vi "HENES.vi"() -> ()   [LabVIEW 2024]
uses:
  <vilib>/Instr/_visa.llb/VISA Set IO Buffer Mask.ctl
  <vilib>/Instr/_visa.llb/VISA Flush IO Buffer Mask.ctl
  e33ea129-5426-40bd-9da2-e127971607b1.vi
  <vilib>/Instr/_visa.llb/VISA Configure Serial Port (Instr).vi
panel:
  out "GobackROI":cluster{i32[], i32[]}={[500, 500, -500, -500, 500], [100, 950, 950, 100, 100]}
  in  "Stop":bool
  in  "탭 컨트롤":enum32{"Main", "Debug"}(tab)
  in  "HLV_A/M":bool=TRUE
  out "Remote_M/A":bool
  out "E-STOP":bool=TRUE
  out "Alive_PCU":u8(slide)=1 scale=0.0..254.0
  out "Speed_Feed(RPM)":dbl format="%#_g rpm"
  in  "HLV_E-stop":bool
  out "Speed_Feed(m/s)":dbl
  in  "Input_Spd(kph)":dbl=7.0
  out "Input_Spd(cmd)":dbl=538.4742241275792
  in  "Lidar Tab":enum32{"Lidar", "Debug"}(tab)
  out "PointCloud":T1(graph)=[{"appended array"=[700.0, 700.0, 3500.0, 3500.0, -3500.0, -3500.0, -700.0, -700.0, 700.0], "appended array"=[800.0, -800.0, -800.0, 5200.0, 5200.0, -800.0, -800.0, 800.0, 800.0]}, {"appended array"=[-450.0], "appended array"=[-250.0]}, {"appended array"=[-450.0, -450.0, -800.0, -800.0, 0.0, 0.0, -450.0], "appended array"=[100.0, -800.0, -800.0, 1200.0, 1200.0, 100.0, 100.0]}, {"appended array"=[800.0, 750.0, 800.0, 800.0, 800.0, 800.0, 800.0], "appended array"=[400.0, 350.0, 350.0, 300.0, 250.0, 200.0, 150.0]}, {"appended array"=[450.0, 450.0, 800.0, 800.0, 0.0, 0.0, 450.0], "appended array"=[100.0, -800.0, -800.0, 1200.0, 1200.0, 100.0, 100.0]}, {"appended array"=array[442 elements], "appended array"=array[442 elements]}, {"appended array"=[4.2861222383783204e-13, 0.0], "appended array"=[7000.0, 0.0]}, {"appended array"=[500.0, 500.0, -500.0, -500.0, 500.0], "appended array"=[100.0, 950.0, 950.0, 100.0, 100.0]}]
  in  "격자크기":dbl=50.0
  out "LidarLoop":u32=101
  in  "Ratio_Threshold":i32=4
  in  "min_samples":i32=2
  in  "eps":i32=100
  in  "Spacing":i32=100
  in  "Threshold":i32=2100
  out "Too Close":bool=TRUE caption="lidar_state"
  in  "Looking Y":i32=5200
  in  "Looking X":i32=3500
  out "Anthena_Steer":i32
  out "NearSteer":dbl=28.559259641865033
  out "TooClose":bool=TRUE
  out "PythonLoop":u32=101
  in  "LiDAR":refnum<visa-resource-name>="COM5"
  in  "GoBack":bool
  out "VEstop":bool
  in  "length":dbl=1300.0
  out "read buffer":string
  out "Clustering Error":errorcluster
  in  "InputSteer(cmd)":dbl=28.559259641865033
  out "Steer_Feed":dbl=-0.28
  in  "HLV_Gear":u8
  out "Gear_Feed":u8=1
  out "HENES Loop Time":u32=48
  in  "HENES":refnum<visa-resource-name>="COM3"
  out "버퍼 읽기":string
  out "TargetDerection":cluster{dbl[], dbl[]}={[4.2861222383783204e-13, 0.0], [7000.0, 0.0]}
  out "NearLeft":dbl=77.70286898858113
  out "NearRight":dbl=-49.1436093467161
  out "Y_arraysREAL":i32[](array[numeric])=[1650, 1650, 1650, 1650, 1650, 1650, 1650, 1650, 1700, 1700, 1700, 1700, 1700, 1700, 1700, 1700, 1700, 1700, 1700, 1750, 1700]
  out "X_arraysREAL":i32[](array[numeric])=[1000, 1050, 1100, 1150, 1200, 1250, 1300, 1350, 1350, 1400, 1450, 1500, 1550, 1600, 1650, 1700, 1750, 1800, 1850, 1850, 1900]
  out "LookingAt":cluster{i32[], i32[]}={[700, 700, 3500, 3500, -3500, -3500, -700, -700, 700], [800, -800, -800, 5200, 5200, -800, -800, 800, 800]}
  out "Too Close":bool=TRUE caption="lidar_state"
  out "NearCarPointsRight":cluster{"ROI_IN_X":dbl[], "ROI_IN_Y":dbl[]}={"ROI_IN_X"=[750.0, 800.0, 800.0, 800.0, 800.0, 800.0], "ROI_IN_Y"=[350.0, 350.0, 300.0, 250.0, 200.0, 150.0]}
  out "NearCarROIRight":cluster{i32[], i32[]}={[450, 450, 800, 800, 0, 0, 450], [100, -800, -800, 1200, 1200, 100, 100]}
  out "Clustered":T2
  out "NearCarROILeft":cluster{i32[], i32[]}={[-450, -450, -800, -800, 0, 0, -450], [100, -800, -800, 1200, 1200, 100, 100]}
  out "NearCarPointsLeft":cluster{"ROI_IN_X":dbl[], "ROI_IN_Y":dbl[]}={"ROI_IN_X"=[-450.0, -550.0], "ROI_IN_Y"=[-250.0, -300.0]}
  out "Y_arrays":dbl[](array[numeric])=[1650.0, 1650.0, 1650.0, 1650.0, 1650.0, 1650.0, 1650.0, 1700.0, 1700.0, 1700.0, 1700.0, 1700.0, 1700.0, 1700.0, 1700.0, 1700.0, 1700.0, 1700.0, 1750.0, 1700.0, 1700.0, 1750.0, 1750.0, 1750.0, 1750.0, 1750.0, 1750.0, 1750.0, 1750.0, 1750.0, 1750.0, 1750.0, 1800.0, 1800.0, 1800.0, 1800.0, 1800.0, 1800.0, 1800.0, 1800.0, 1800.0, 1800.0, 1800.0, 1800.0, 1800.0, 1800.0, 1800.0, 1800.0, 1800.0, 1850.0, 1850.0, 1850.0, 350.0, 350.0, 350.0, 300.0, 250.0, 200.0, 200.0, 150.0, 150.0, 100.0, 50.0, 0.0, -50.0, -100.0, -150.0, -200.0, -250.0, -300.0, -300.0, -350.0, -400.0, -450.0, -500.0, -550.0, -600.0, -650.0, -700.0, -750.0, -800.0, -800.0, -750.0, -750.0, -700.0, -700.0, -650.0, -600.0, -550.0, -550.0, -500.0, -450.0, -400.0, -350.0, -300.0, -250.0, -200.0, -150.0, -100.0, -50.0, 0.0, 50.0, 100.0, 150.0, 200.0, 250.0, 300.0, 350.0, 400.0, 400.0, 450.0, 500.0, 550.0, 600.0, 600.0, 650.0, 650.0, 700.0, 700.0, 750.0, 750.0, 800.0, 800.0, 850.0, 850.0, 900.0, 900.0, 950.0, 950.0, 1000.0, 1000.0, 1050.0, 1050.0, 1100.0, 1100.0, 1150.0, 1150.0, 1200.0, 1200.0, 1250.0, 1250.0, 1300.0, 1300.0, 1350.0, 1400.0, 1450.0, 1500.0, 1550.0, 1600.0, 1650.0, 1700.0, 1750.0, 1800.0, 1850.0, 1900.0, 1950.0, 2000.0, 2050.0, 2100.0, 2150.0, 2200.0, 2250.0, 2300.0, 2350.0, 2400.0, 2450.0, 2500.0, 2550.0, 2600.0, 2600.0, 2650.0, 2700.0, 2750.0, 2800.0, 2850.0, 2900.0, 2950.0, 3000.0, 3050.0, 3100.0, 3150.0, 3200.0, 3250.0, 3300.0, 3350.0, 3400.0, 3450.0, 3450.0, 3500.0, 3550.0, 3600.0, 3650.0, 3700.0, 3750.0, 3800.0, 3850.0, 3900.0, 3950.0, 4000.0, 4000.0, 4100.0, 4150.0, 4200.0, 4250.0, 4300.0, 4350.0, 4400.0, 4450.0, 4500.0, 4550.0, 4600.0, 4650.0, 4700.0, 4750.0, 4800.0, 4900.0, 4950.0, 5000.0, 5050.0, 5100.0, 5150.0, 4500.0, 4500.0, 4600.0, 4550.0, 3800.0, 3700.0, 3650.0, 3600.0, 3550.0, 3500.0, 3500.0, 3450.0, 3400.0, 3350.0, 3300.0, 3250.0, 3250.0, 3200.0, 3150.0, 3200.0, 3200.0, 3200.0, 3400.0, 3450.0, 3200.0, 4700.0, 4700.0, 3700.0, 3450.0, 3400.0, 3450.0, 3500.0, 3500.0, 3450.0, 3400.0, 3400.0, 3350.0, 3300.0, 3300.0, 3250.0, 1600.0, 1600.0, 1650.0, 1600.0, 1650.0, 1735.0877192982457, -160.3448275862069, 1825.7462686567164, 5025.0, 4500.0, 4575.0, 3392.1052631578946, 3425.0, 4700.0, 3395.8333333333335, 1827.3513645224173, 1919.6150097465888, 2011.8786549707602, 2104.142300194932, 2196.4059454191033, 2288.669590643275, 2380.9332358674465, 2473.196881091618, 2565.4605263157896, 2657.7241715399614, 2749.9878167641327, 2842.251461988304, 2934.5151072124754, 3026.778752436647, 3119.042397660819, 3211.3060428849903, 3303.5696881091617, 1824.0304709141276, 1912.9732225300093, 2001.9159741458911, 2090.858725761773, 2179.801477377655, 2268.7442289935366, 2357.6869806094182, 2446.6297322253004, 2535.572483841182, 2624.5152354570637, 2713.457987072946, 2802.400738688827, 2891.343490304709, 2980.2862419205912, 3069.228993536473, 3158.1717451523546, 3247.114496768236, 3336.057248384118, 1817.938596491228, 1900.7894736842106, 1983.640350877193, 2066.4912280701756, 2149.342105263158, 2232.1929824561403, 2315.043859649123, 2397.8947368421054, 2480.745614035088, 2563.59649122807, 2646.4473684210525, 2729.2982456140353, 2812.149122807017, 2895.0, 2977.8508771929824, 3060.7017543859647, 3143.5526315789475, 3226.4035087719294, 3309.254385964912, 4515.0, 4530.0, 4545.0, 4560.0, 4407.675438596491, 4315.350877192983, 4223.026315789473, 4130.701754385965, 4038.377192982456, 3946.0526315789475, 3853.7280701754385, 3761.40350877193, 3669.078947368421, 3576.754385964912, 3484.4298245614036, 4417.307692307692, 4334.615384615385, 4251.923076923077, 4169.2307692307695, 4086.5384615384614, 4003.846153846154, 3921.153846153846, 3838.4615384615386, 3755.769230769231, 3673.076923076923, 3590.3846153846152, 3507.6923076923076, 4588.888888888889, 4602.777777777777, 4616.666666666667, 4630.555555555556, 4644.444444444444, 4658.333333333333, 4672.222222222223, 4686.111111111111, 4479.166666666667, 4383.333333333333, 4287.5, 4191.666666666667, 4095.8333333333335, 4000.0, 3904.166666666667, 3808.3333333333335, 3712.5, 3616.666666666667, 3520.8333333333335, 3403.0701754385964, 3414.035087719298, 3392.6378446115286, 3393.1704260651627, 3393.7030075187968, 3394.2355889724313, 3394.7681704260654, 3395.3007518796994, 3417.7083333333335, 3410.416666666667, 3403.125, 4684.615384615385, 4669.2307692307695, 4653.846153846154, 4638.461538461538, 4623.076923076923, 4607.692307692308, 4592.307692307692, 4576.923076923077, 4561.538461538462, 4546.153846153846, 4530.7692307692305, 4515.384615384615, 4606.8452380952385, 4513.690476190476, 4420.535714285715, 4327.380952380952, 4234.226190476191, 4141.071428571428, 4047.916666666667, 3954.761904761905, 3861.607142857143, 3768.452380952381, 3675.2976190476193, 3582.1428571428573, 3488.9880952380954, 3486.538461538462, 3577.24358974359, 3667.9487179487182, 3758.653846153846, 3849.3589743589746, 3940.0641025641025, 4030.769230769231, 4121.474358974359, 4212.179487179487, 4302.884615384615, 4393.589743589744, 4484.294871794872]
  out "X_arrays":dbl[](array[numeric])=[1050.0, 1100.0, 1150.0, 1200.0, 1250.0, 1300.0, 1350.0, 1350.0, 1400.0, 1450.0, 1500.0, 1550.0, 1600.0, 1650.0, 1700.0, 1750.0, 1800.0, 1850.0, 1850.0, 1900.0, 1950.0, 2000.0, 2050.0, 2100.0, 2150.0, 2200.0, 2250.0, 2300.0, 2350.0, 2400.0, 2450.0, 2500.0, 2500.0, 2550.0, 2600.0, 2650.0, 2700.0, 2750.0, 2800.0, 2850.0, 2900.0, 2950.0, 3000.0, 3050.0, 3100.0, 3150.0, 3200.0, 3250.0, 3300.0, 3350.0, 3400.0, 3450.0, 750.0, 800.0, 850.0, 800.0, 800.0, 800.0, 850.0, 800.0, 850.0, 850.0, 850.0, 850.0, 850.0, 850.0, 850.0, 850.0, 850.0, 850.0, 900.0, 900.0, 900.0, 900.0, 900.0, 900.0, 900.0, 900.0, 900.0, 900.0, 900.0, -2250.0, -2250.0, -2300.0, -2300.0, -2250.0, -2300.0, -2300.0, -2300.0, -2350.0, -2300.0, -2300.0, -2300.0, -2300.0, -2300.0, -2300.0, -2300.0, -2300.0, -2300.0, -2300.0, -2300.0, -2300.0, -2300.0, -2300.0, -2300.0, -2300.0, -2300.0, -2300.0, -2250.0, -2300.0, -2300.0, -2300.0, -2300.0, -2300.0, -2250.0, -2250.0, -2300.0, -2250.0, -2300.0, -2300.0, -2250.0, -2300.0, -2250.0, -2300.0, -2250.0, -2300.0, -2250.0, -2250.0, -2300.0, -2300.0, -2250.0, -2250.0, -2300.0, -2250.0, -2300.0, -2250.0, -2300.0, -2250.0, -2300.0, -2300.0, -2250.0, -2300.0, -2250.0, -2250.0, -2250.0, -2250.0, -2250.0, -2250.0, -2250.0, -2250.0, -2250.0, -2250.0, -2250.0, -2250.0, -2250.0, -2250.0, -2250.0, -2250.0, -2250.0, -2250.0, -2250.0, -2250.0, -2250.0, -2250.0, -2250.0, -2250.0, -2250.0, -2250.0, -2250.0, -2300.0, -2300.0, -2300.0, -2300.0, -2300.0, -2300.0, -2300.0, -2300.0, -2300.0, -2300.0, -2300.0, -2300.0, -2300.0, -2300.0, -2300.0, -2300.0, -2300.0, -2300.0, -2350.0, -2350.0, -2350.0, -2350.0, -2350.0, -2350.0, -2350.0, -2350.0, -2350.0, -2350.0, -2350.0, -2350.0, -2400.0, -2400.0, -2400.0, -2400.0, -2400.0, -2400.0, -2400.0, -2400.0, -2400.0, -2400.0, -2400.0, -2400.0, -2400.0, -2400.0, -2400.0, -2400.0, -2450.0, -2450.0, -2450.0, -2450.0, -2450.0, -2450.0, 650.0, 700.0, 1100.0, 1150.0, 950.0, 950.0, 950.0, 950.0, 950.0, 950.0, 1000.0, 1000.0, 1000.0, 1000.0, 1000.0, 1000.0, 1050.0, 1050.0, 1050.0, 1100.0, 1150.0, 1200.0, 1300.0, 1350.0, 1250.0, 1900.0, 1950.0, 1600.0, 1500.0, 1550.0, 1600.0, 1600.0, 1650.0, 1650.0, 1650.0, 1700.0, 1650.0, 1650.0, 1700.0, 1700.0, 900.0, 950.0, 950.0, 1000.0, 1000.0, 2118.4210526315787, 856.8965517241379, -2300.0, -2450.0, 675.0, 1125.0, 1028.9473684210527, 1325.0, 1925.0, 1633.3333333333333, 2091.4717348927875, 2064.522417153996, 2037.5730994152045, 2010.623781676413, 1983.6744639376216, 1956.7251461988303, 1929.7758284600388, 1902.8265107212474, 1875.877192982456, 1848.9278752436646, 1821.9785575048732, 1795.029239766082, 1768.0799220272904, 1741.130604288499, 1714.1812865497075, 1687.231968810916, 1660.2826510721247, 2076.6620498614957, 2034.9030470914126, 1993.1440443213294, 1951.3850415512463, 1909.6260387811633, 1867.8670360110802, 1826.108033240997, 1784.349030470914, 1742.590027700831, 1700.8310249307478, 1659.0720221606648, 1617.3130193905818, 1575.5540166204987, 1533.7950138504154, 1492.0360110803324, 1450.2770083102494, 1408.5180055401663, 1366.759002770083, 2063.9473684210525, 2009.4736842105262, 1954.9999999999998, 1900.5263157894735, 1846.0526315789473, 1791.5789473684208, 1737.1052631578946, 1682.6315789473683, 1628.157894736842, 1573.6842105263158, 1519.2105263157894, 1464.736842105263, 1410.2631578947367, 1355.7894736842104, 1301.3157894736842, 1246.842105263158, 1192.3684210526317, 1137.8947368421054, 1083.421052631579, 765.0, 855.0, 945.0, 1035.0, 704.4956140350878, 733.9912280701755, 763.4868421052631, 792.9824561403509, 822.4780701754387, 851.9736842105264, 881.469298245614, 910.9649122807018, 940.4605263157896, 969.9561403508773, 999.4517543859649, 725.0, 775.0, 825.0, 875.0, 925.0, 975.0, 1025.0, 1075.0, 1125.0, 1175.0, 1225.0, 1275.0, 1213.888888888889, 1302.7777777777778, 1391.6666666666665, 1480.5555555555557, 1569.4444444444443, 1658.3333333333333, 1747.2222222222222, 1836.111111111111, 1141.6666666666667, 1158.3333333333333, 1175.0, 1191.6666666666667, 1208.3333333333333, 1225.0, 1241.6666666666667, 1258.3333333333333, 1275.0, 1291.6666666666667, 1308.3333333333333, 1127.6315789473686, 1226.3157894736842, 1115.2882205513786, 1201.6290726817042, 1287.96992481203, 1374.310776942356, 1460.6516290726815, 1546.9924812030074, 1402.0833333333333, 1479.1666666666665, 1556.25, 1828.8461538461538, 1732.6923076923076, 1636.5384615384614, 1540.3846153846152, 1444.2307692307693, 1348.076923076923, 1251.9230769230767, 1155.7692307692307, 1059.6153846153848, 963.4615384615385, 867.3076923076922, 771.1538461538462, 1904.1666666666667, 1883.3333333333333, 1862.5, 1841.6666666666667, 1820.8333333333333, 1800.0, 1779.1666666666665, 1758.3333333333333, 1737.5, 1716.6666666666665, 1695.8333333333333, 1675.0, 1654.1666666666665, 1594.230769230769, 1555.128205128205, 1516.0256410256409, 1476.923076923077, 1437.8205128205127, 1398.7179487179487, 1359.6153846153845, 1320.5128205128203, 1281.4102564102564, 1242.3076923076924, 1203.2051282051282, 1164.102564102564]
  out "Y_arrays_input":i32[](array[numeric])=[1650, 1650, 1650, 1650, 1650, 1650, 1650, 1650, 1700, 1700, 1700, 1700, 1700, 1700, 1700, 1700, 1700, 1700, 1700, 1750, 1700]
  out "X_arrays_input":i32[](array[numeric])=[1000, 1050, 1100, 1150, 1200, 1250, 1300, 1350, 1350, 1400, 1450, 1500, 1550, 1600, 1650, 1700, 1750, 1800, 1850, 1850, 1900]
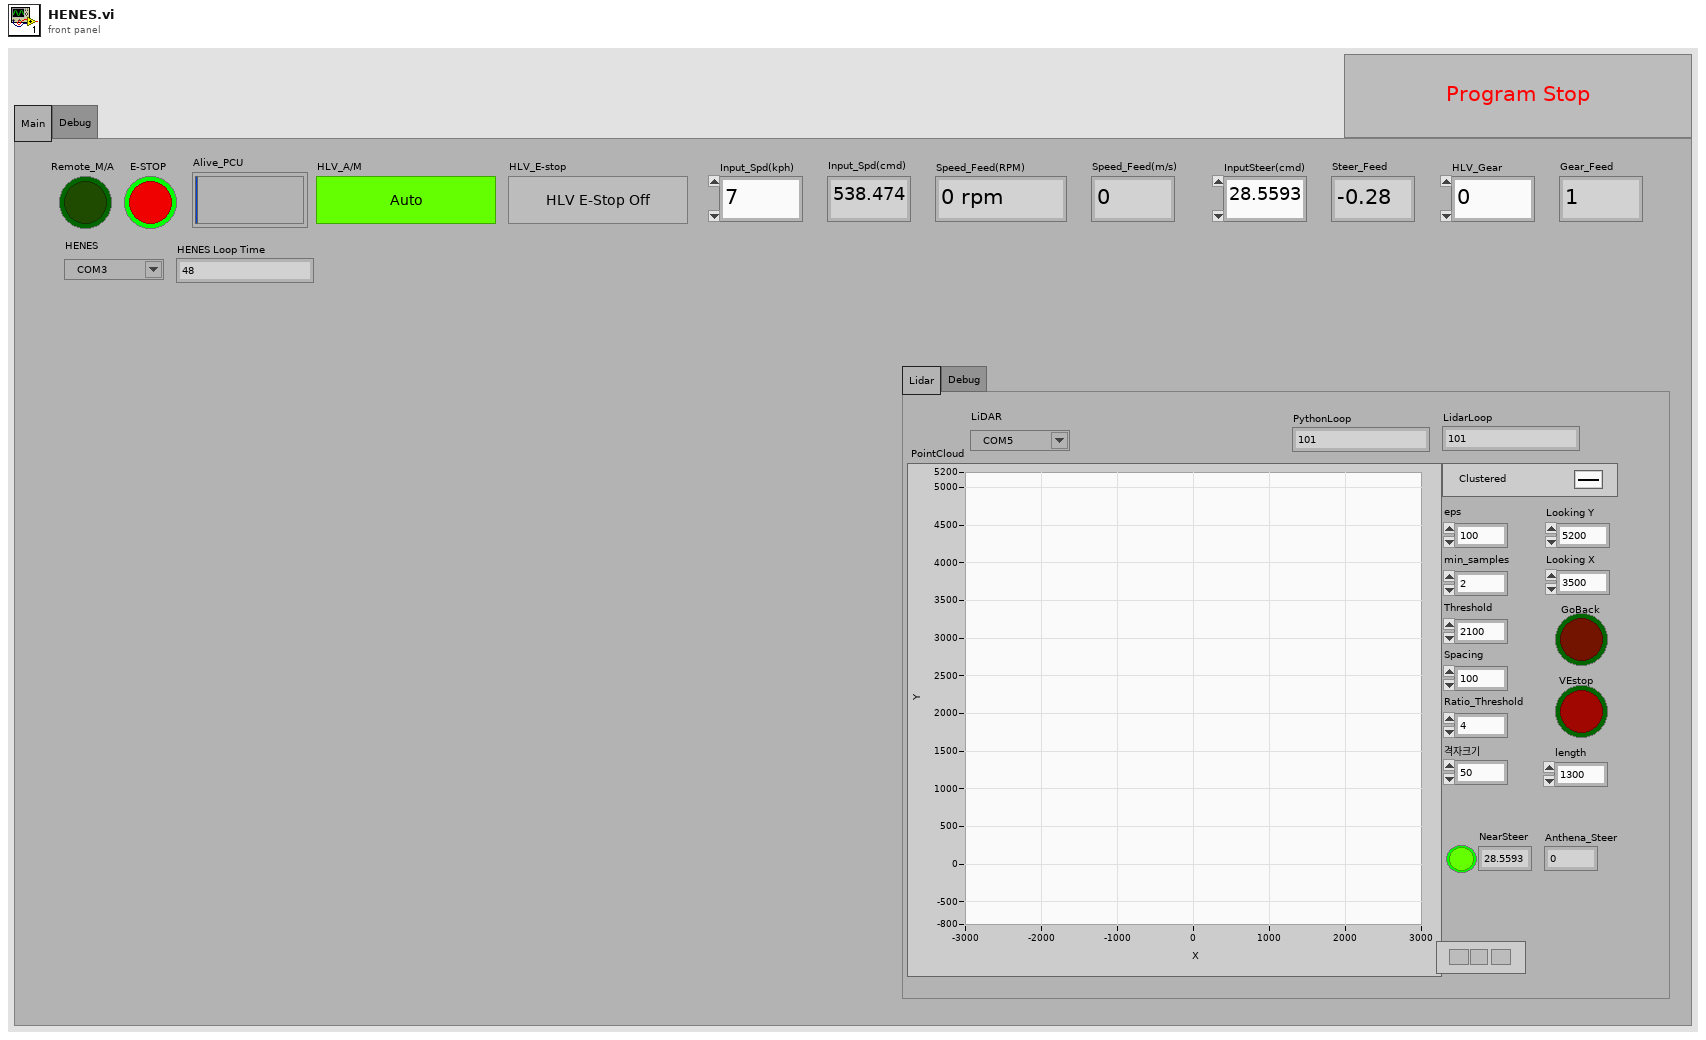
[diagram p1: front panel]
types:
  T1 = cluster{"appended array":dbl[], "appended array":dbl[]}[]
  T2 = cluster{"appended array":dbl[], "appended array":dbl[]}
  T3 = cluster{"HENES_M/A":u8, "HENES_E-Stop":u8, "HENES_Gear":u8, "HENES_Speed":i16, "HENES_Steer":i16, "HENES_Alive":u8}
  T4 = typedef "VISA Flush IO Buffer Mask.ctl" = u16
  T5 = typedef "VISA Set IO Buffer Mask.ctl" = u16
  T6 = cluster{"HLV_M/A_Status":u8, "HLV_E-Stop":u8, "HLV_Gear":u8, "HLV_Speed":i16, "HLV_Steer":i16, "HLV_Alive":u8}
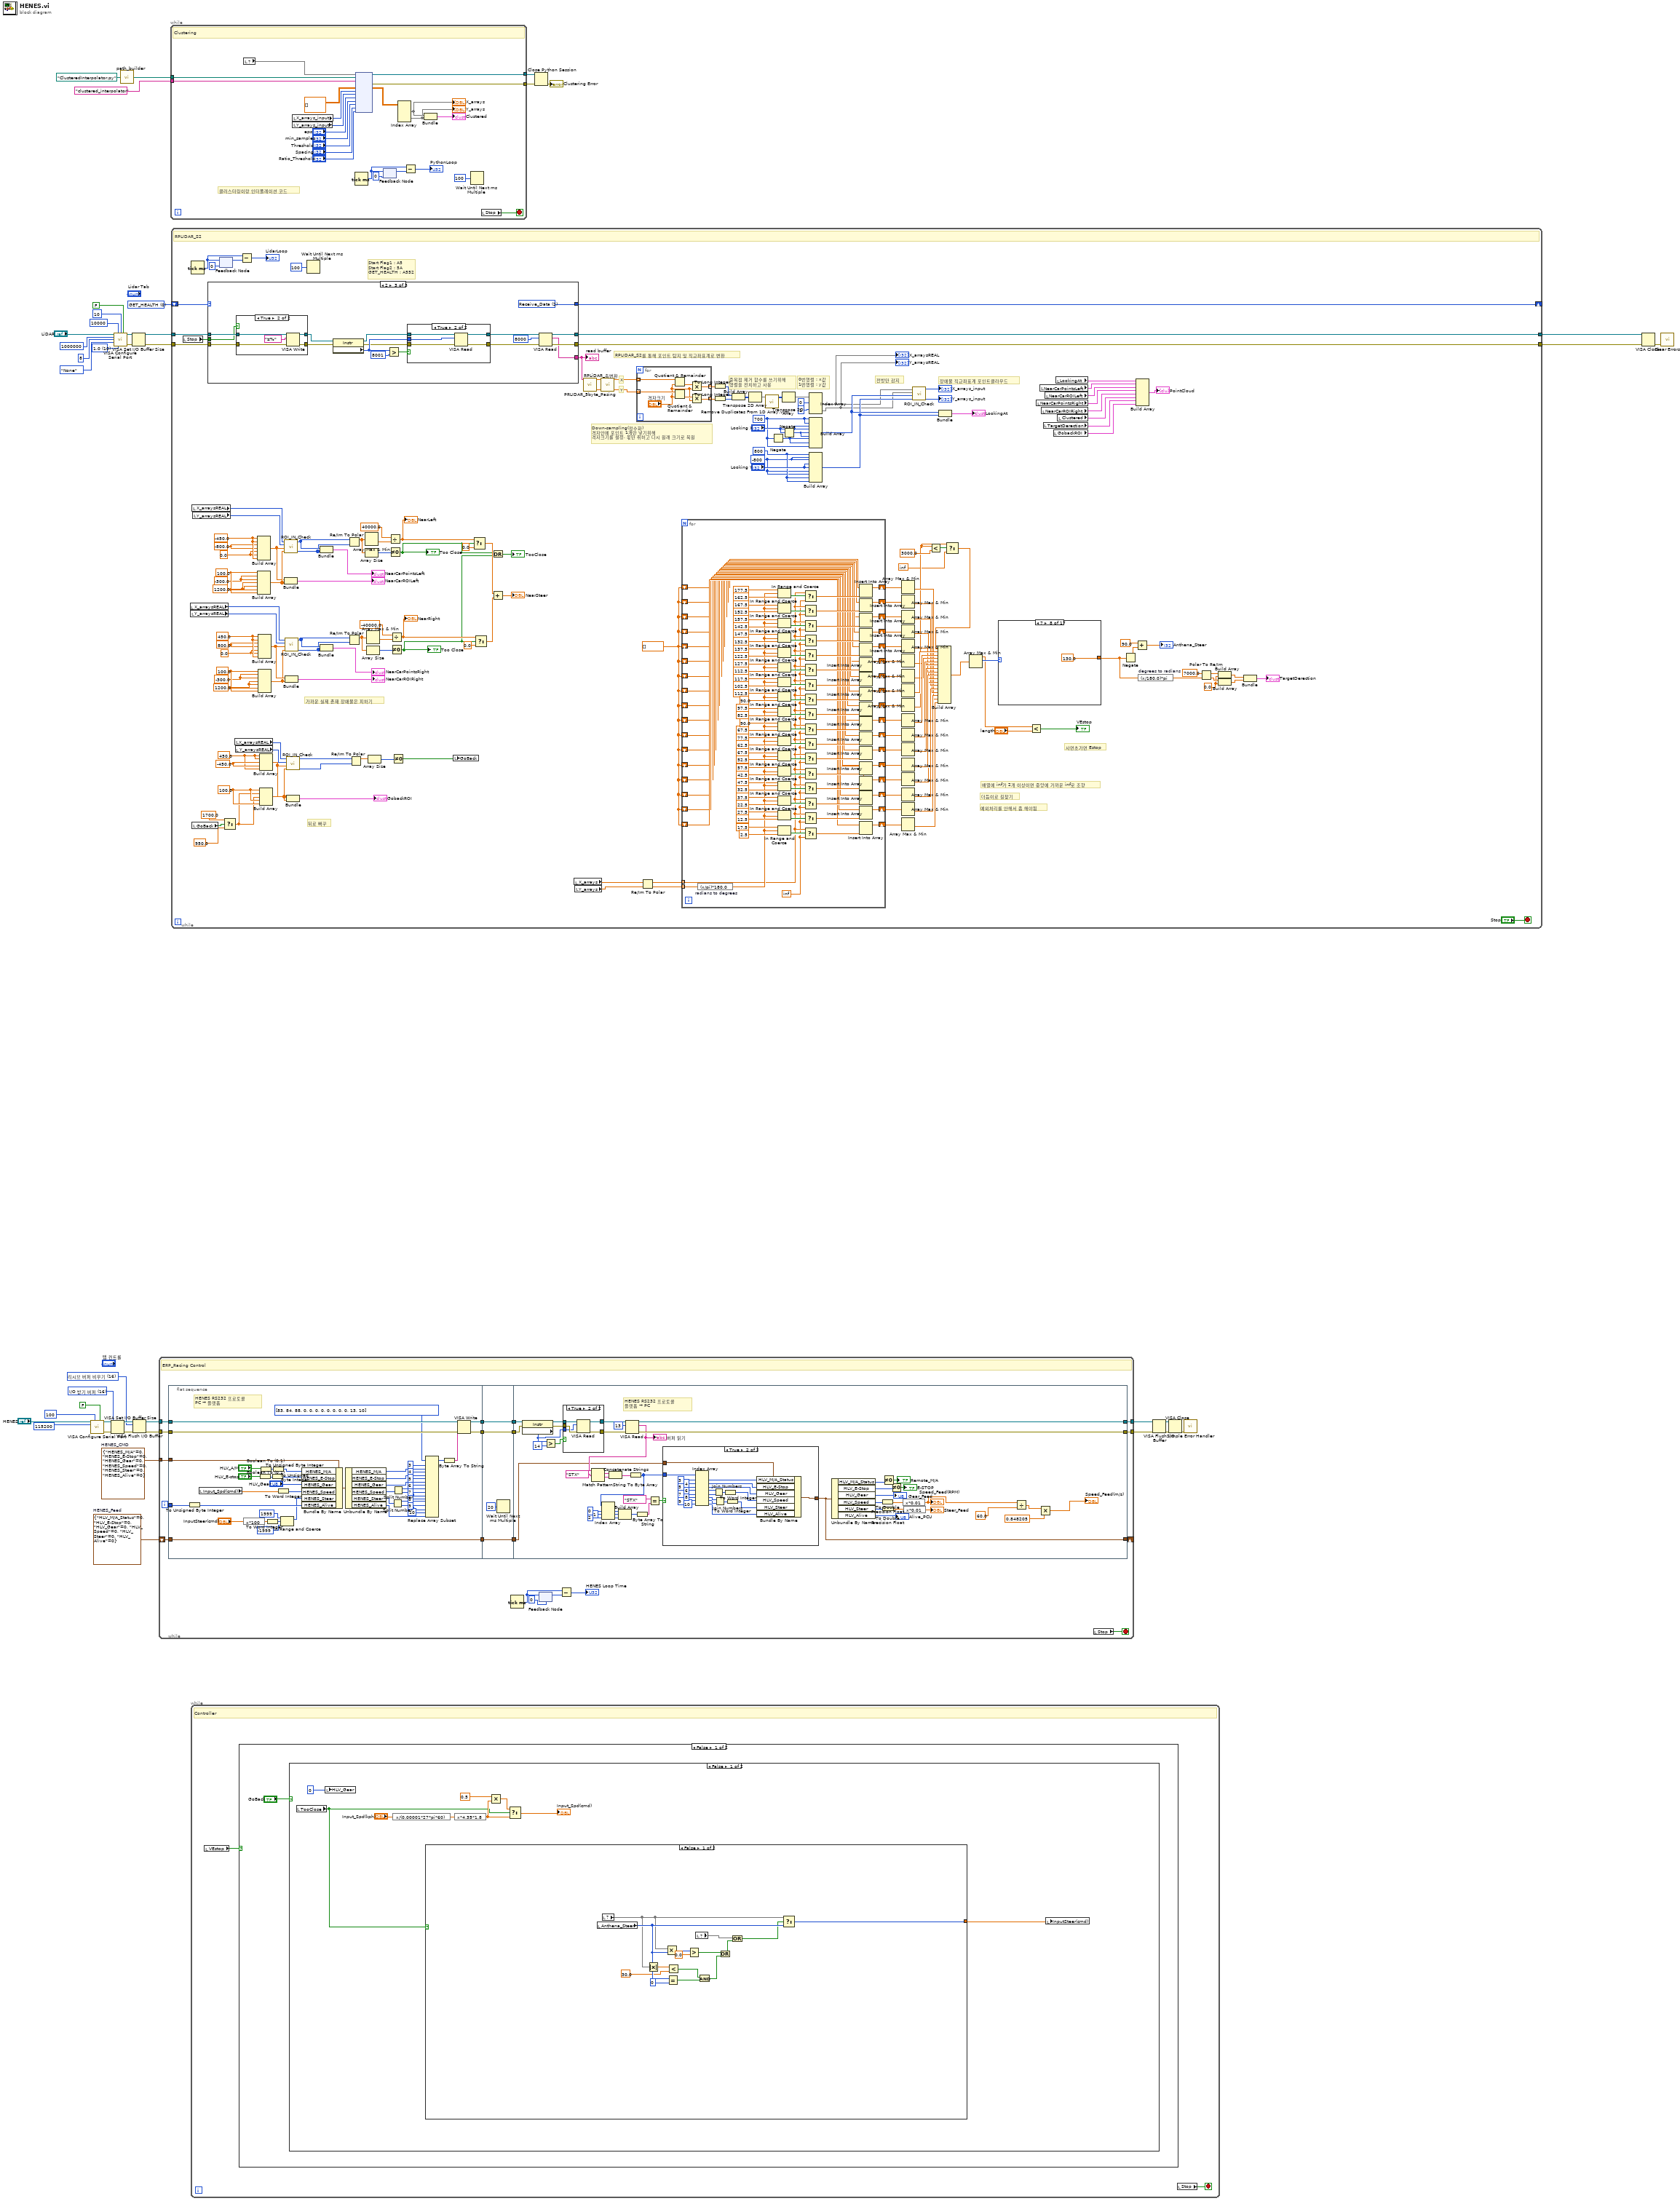
[diagram p0: block diagram]
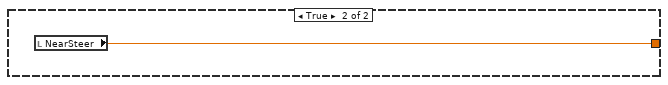
[diagram p2: hidden frame]
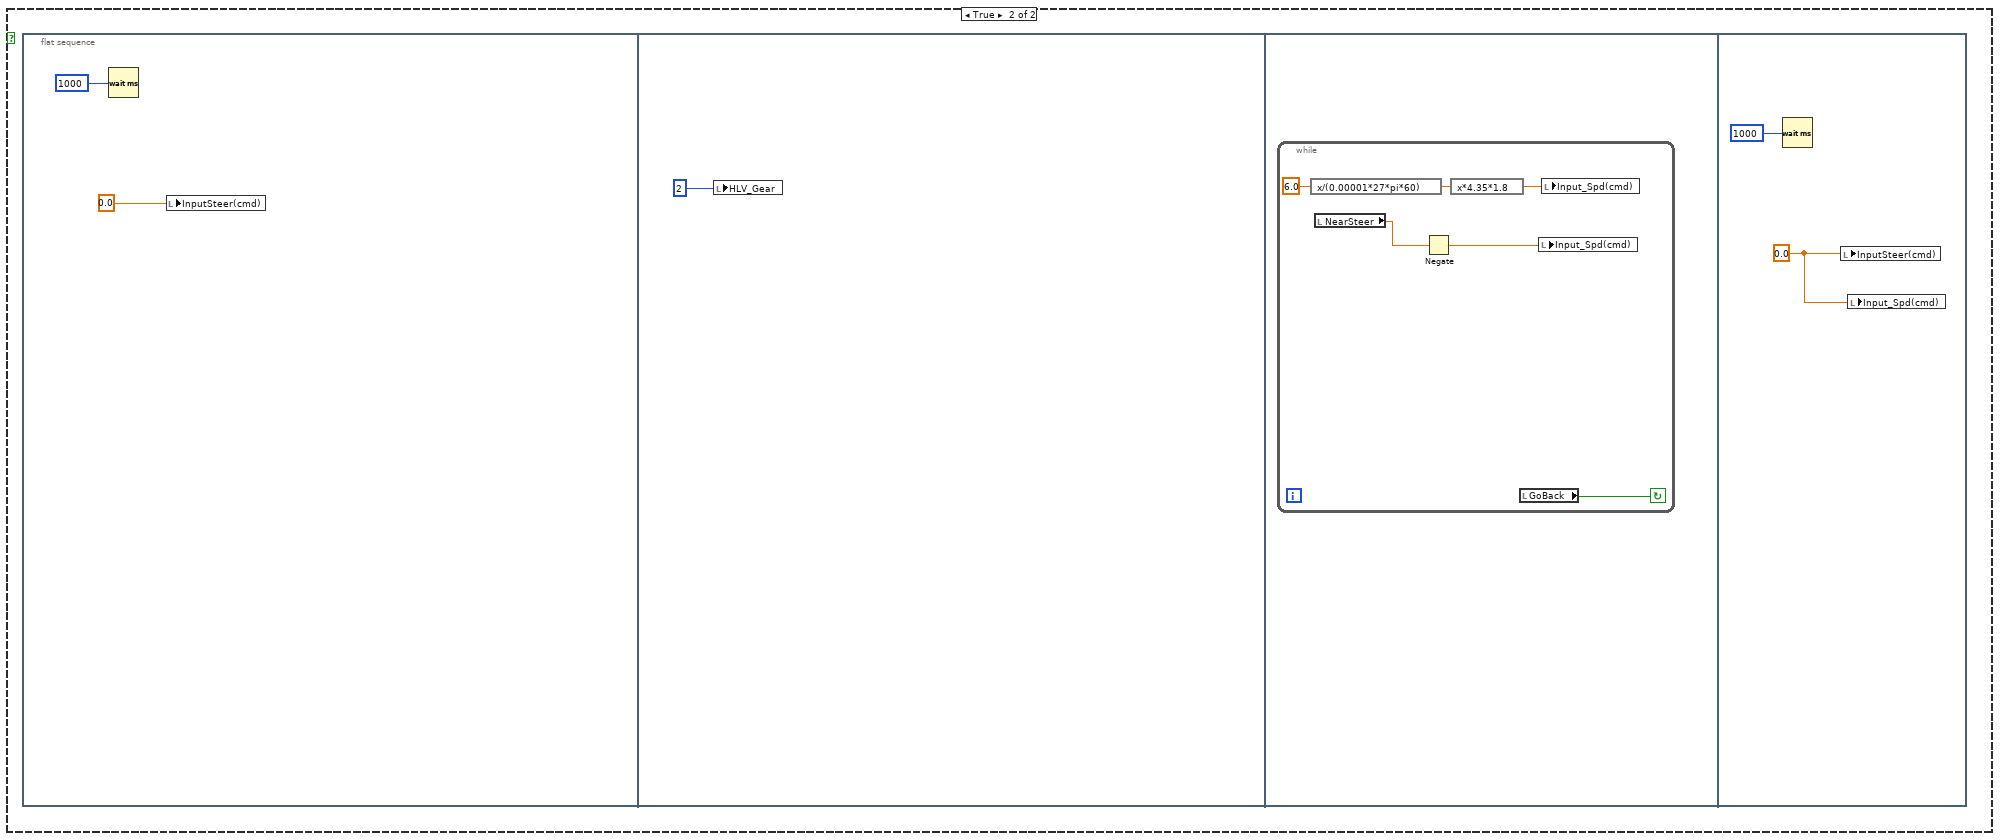
[diagram p3: hidden frame]
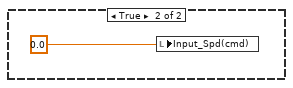
[diagram p4: hidden frame]
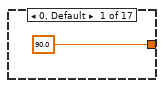
[diagram p7: hidden frame]
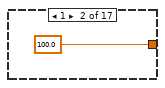
[diagram p8: hidden frame]
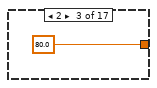
[diagram p9: hidden frame]
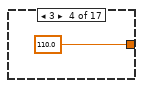
[diagram p10: hidden frame]
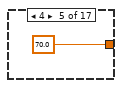
[diagram p11: hidden frame]
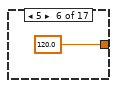
[diagram p12: hidden frame]
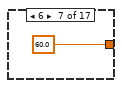
[diagram p13: hidden frame]
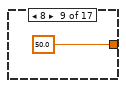
[diagram p14: hidden frame]
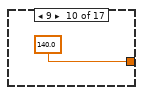
[diagram p15: hidden frame]
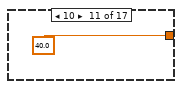
[diagram p16: hidden frame]
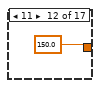
[diagram p17: hidden frame]
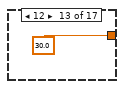
[diagram p18: hidden frame]
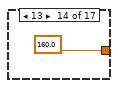
[diagram p19: hidden frame]
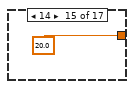
[diagram p20: hidden frame]
diagram:
  w3 = T3 {"HENES_M/A"=0, "HENES_E-Stop"=0, "HENES_Gear"=0, "HENES_Speed"=0, "HENES_Steer"=0, "HENES_Alive"=0}  # HENES_CMD
  w6 = T4 16 items=["리시브 버퍼 비우기"=16, "전달 버퍼 디바이스에 쓰기"=32, "리시브 버퍼 비우기(I/O 없음)"=64, "전달 버퍼 비우기"=128] ("Mask")
  w9 = T5 16 items=["I/O 받기 버퍼"=16, "I/O 전달 버퍼"=32, "I/O 받기와 전달 버퍼"=48] ("Mask")
  w13 = T6 {"HLV_M/A_Status"=0, "HLV_E-Stop"=0, "HLV_Gear"=0, "HLV_Speed"=0, "HLV_Steer"=0, "HLV_Alive"=0}  # HENES_Feed
  w27 = u16 10 items=["1.0"=10, "1.5"=15, "2.0"=20] ("stop bits (10: 1 bit)")
  w29 = u16 0 items=["GET_HEALTH", "SCAN_START", "Receive_Data"]
  n1 = call-poly "VISA Configure Serial Port"("VISA resource name"="HENES", "timeout (10sec)"=u32 100, "Enable Termination\nChar (T)"=FALSE ("Enable Termination\nChar (T)"), "baud rate (9600)"=u32 115200) -> ("VISA resource name out"=w5:refnum<visa-resource-name>, "error out"=w4:errorcluster)  [unwired: 10 in]
  n2 = VISA Set I/O Buffer Size(VISA resource name=w5, mask (16)=w9, error in (no error)=w4) -> (VISA resource name out=w8:refnum<visa-resource-name>, error out=w7:errorcluster)  [unwired: 1 in]
  n3 = call-poly "VISA Configure Serial Port"("VISA resource name"="LiDAR", "timeout (10sec)"=u32 10000, "termination char\n(0xA = '\\n' = LF)"=u8 10 ("termination char\n(0xA = '\\n' = LF)"), "Enable Termination\nChar (T)"=FALSE ("Enable Termination\nChar (T)"), "baud rate (9600)"=u32 1000000, "data bits (8)"=u16 8, "parity (0:none)"=enum16{"None", "Odd", "Even", "Mark", "Space"}."None", "stop bits (10: 1 bit)"=w27) -> ("VISA resource name out"=w36:refnum<visa-resource-name>, "error out"=w35:errorcluster)  [unwired: 6 in]
  n4 = call "path_builder.vi"("Name"=path "ClusteredInterpolator.py") -> ("appended path"=w22:path)
  n5 = VISA Set I/O Buffer Size(VISA resource name=w36, error in (no error)=w35) -> (VISA resource name out=w31:refnum<visa-resource-name>, error out=w30:errorcluster)  [unwired: 2 in]
  n6 = VISA Flush I/O Buffer(VISA resource name=w8, mask (16)=w6, error in (no error)=w7) -> (VISA resource name out=w18:refnum<visa-resource-name>, error out=w17:errorcluster)
  n7 = while {
    tunnel: w18 -> [w60]
    tunnel: w17 -> [w59]
    tunnel: [w53] -> w16
    tunnel: [w52] -> w15
    shift-right: [w47] -> _
    shift-left: w13 -> [w50]
    tunnel: w3 -> [w48]
    i -> [w54]
    stop <- w42 stop-if-true
    # "ERP_Racing Control"
    n8 = flat-sequence {
      tunnel: [w103] -> w57
      tunnel: [w102] -> w55
      tunnel: w60 -> [w105]
      tunnel: w59 -> [w104]
      tunnel: w54 -> [w101]
      tunnel: [w100] -> w51
      tunnel: w50 -> [w100]
      tunnel: w48 -> [w99]
      tunnel: [w109] -> w58
      tunnel: w57 -> [w109]
      tunnel: [w108] -> w56
      tunnel: w55 -> [w108]
      tunnel: w51 -> [w106]
      tunnel: [w106] -> w49
      tunnel: w58 -> [w137]
      tunnel: w56 -> [w136]
      tunnel: [w154] -> w53
      tunnel: [w153] -> w52
      tunnel: w49 -> [w128]
      tunnel: [w126] -> w47
      frame #0 {
        # "HENES RS232 프로토콜\nPC → 플랫폼"
        n9 = To Unsigned Byte Integer(number=w101) -> (unsigned 8bit integer=w88:u8)
        n10 = local read "Input_Spd(cmd)"() -> (w62:dbl)
        n11 = expression code="x*100"("InputSteer(cmd)") -> (w63:dbl)
        n12 = Boolean To (0,1)(Boolean="HLV_E-stop") -> (0, 1=w83:i16)
        n13 = Boolean To (0,1)(Boolean="HLV_A/M") -> (0, 1=w84:i16)
        n14 = To Word Integer(number=w63) -> (16bit integer=w66:i16)
        n15 = To Unsigned Byte Integer(number=w83) -> (unsigned 8bit integer=w81:u8)
        n16 = To Unsigned Byte Integer(number=w84) -> (unsigned 8bit integer=w82:u8)
        n17 = To Word Integer(number=w62) -> (16bit integer=w75:i16)
        n18 = In Range and Coerce(upper limit=i16 1999 ("상위 리미트"), x=w66, lower limit=i16 -1999 ("상위 리미트")) -> (coerced(x)=w74:i16)  [unwired: 1 out]
        n19 = Bundle By Name(cluster=w99, "HENES_M/A"=w82, "HENES_E-Stop"=w81, "HENES_Gear"="HLV_Gear", "HENES_Speed"=w75, "HENES_Steer"=w74, "HENES_Alive"=w88) -> (w92:T3)
        n20 = Unbundle By Name(w92) -> ("HENES_M/A"=w78:u8, "HENES_E-Stop"=w77:u8, "HENES_Gear"=w67:u8, "HENES_Speed"=w70:i16, "HENES_Steer"=w73:i16, "HENES_Alive"=w87:u8)
        n21 = Split Number(x=w73) -> (hi(x)=w72:u8, lo(x)=w71:u8)
        n22 = Split Number(x=w70) -> (hi(x)=w69:u8, lo(x)=w68:u8)
        n23 = Replace Array Subset(array=u8[] [83, 84, 88, 0, 0, 0, 0, 0, 0, 0, 0, 13, 10] ("unsigned byte array"), new element #1=w78, index #1=3, new element #2=w77, index #2=4, new element #3=w67, index #3=5, new element #4=w69, index #4=6, new element #5=w68, index #5=7, new element #6=w72, index #6=8, new element #7=w71, index #7=9, new element #8=w87, index #8=10) -> (w90:u8[])
        n24 = Byte Array To String(unsigned byte array=w90) -> (string=w89:string)
        n25 = VISA Write(VISA resource name=w105, write buffer=w89, error in (no error)=w104) -> (VISA resource name out=w103:refnum<visa-resource-name>, error out=w102:errorcluster)  [unwired: 1 out]
      }
      frame #1 {
        n26 = Wait Until Next ms Multiple(millisecond multiple=u32 20 ("대기 시간 (ms)")) -> ()  [unwired: 1 out]
      }
      frame #2 {
        # "HENES RS232 프로토콜\n플랫폼 → PC"
        n27 = property class="Instr"(reference=w137, error in=w136) -> (reference out=w117:refnum<visa-resource-name>, error out=w116:errorcluster, "Serial Settings:Number of Bytes at Serial Port"=w115:u32)
        n28 = Greater?(x=w115, y=u32 14) -> (0:w133:bool)
        n29 = case shown="True" w133 {
          tunnel: w117 -> [w181 w186]
          tunnel: w116 -> [w180 w185]
          tunnel: [w181 w184] -> w135
          tunnel: [w180 w183] -> w134
          tunnel: w115 -> [_ w182]
          frame False {
          }
          frame True {
            n30 = VISA Read(VISA resource name=w186, byte count=w182, error in (no error)=w185) -> (VISA resource name out=w184:refnum<visa-resource-name>, error out=w183:errorcluster)  [unwired: 2 out]
          }
        }
        n31 = VISA Read(VISA resource name=w135, byte count=u32 13, error in (no error)=w134) -> (VISA resource name out=w154:refnum<visa-resource-name>, read buffer=w152:string, error out=w153:errorcluster)  [unwired: 1 out]
        "버퍼 읽기" <- w152
        n32 = Match Pattern(string=w152, regular expression="STX") -> (match substring=w149:string, after substring=w150:string)  [unwired: 1 in, 2 out]
        n33 = Concatenate Strings(w149, w150) -> (w148:string)
        n34 = String To Byte Array(string=w148) -> (unsigned byte array=w130:u8[])
        n35 = Index Array(array=w130, index #1=0, index #2=1, index #3=2) -> (element #1=w143:u8, element #2=w142:u8, element #3=w141:u8)
        n36 = Build Array(w143, w142, w141) -> (w140:u8[])
        n37 = Byte Array To String(unsigned byte array=w140) -> (string=w138:string)
        n38 = Equal?(x="STX", y=w138) -> (x = y?=w129:bool)
        n39 = case shown="True" w129 {
          tunnel: w130 -> [_ w179]
          tunnel: [w156 w166] -> w126
          tunnel: w128 -> [w156 w168]
          frame False {
          }
          frame True {
            n40 = Index Array(array=w179, index #1=3, index #2=4, index #3=5, index #4=6, index #5=7, index #6=8, index #7=9, index #8=10) -> (element #1=w167:u8, element #2=w165:u8, element #3=w164:u8, element #4=w163:u8, element #5=w162:u8, element #6=w160:u8, element #7=w159:u8, element #8=w157:u8)
            n41 = Join Numbers(hi=w163, lo=w162) -> ((hi.lo)=w170:u16)
            n42 = Join Numbers(hi=w160, lo=w159) -> ((hi.lo)=w169:u16)
            n43 = To Word Integer(number=w170) -> (16bit integer=w161:i16)
            n44 = To Word Integer(number=w169) -> (16bit integer=w158:i16)
            n45 = Bundle By Name(cluster=w168, "HLV_M/A_Status"=w167, "HLV_E-Stop"=w165, "HLV_Gear"=w164, "HLV_Speed"=w161, "HLV_Steer"=w158, "HLV_Alive"=w157) -> (w166:T6)
          }
        }
        n46 = Unbundle By Name(w126) -> ("HLV_M/A_Status"=w127:u8, "HLV_E-Stop"=w121:u8, "HLV_Gear"=→"Gear_Feed":u8, "HLV_Speed"=w119:i16, "HLV_Steer"=w118:i16, "HLV_Alive"=→"Alive_PCU":u8)
        n47 = To Double Precision Float(number=w119) -> (double precision float=w131:dbl)
        n48 = To Double Precision Float(number=w118) -> (double precision float=w124:dbl)
        n49 = Not Equal To 0?(x=w127) -> (x != 0?=→"Remote_M/A":bool)
        n50 = Not Equal To 0?(x=w121) -> (x != 0?=→"E-STOP":bool)
        n51 = expression code="x*0.01"(w131) -> (w110:dbl)
        "Speed_Feed(RPM)" <- w110
        n52 = expression code="x*0.01"(w124) -> (→"Steer_Feed":dbl)
        n53 = Divide(x=w110, y=60.0) -> (x/y=w114:dbl)
        n54 = Multiply(x=w114, y=0.848205) -> (x*y=→"Speed_Feed(m/s)":dbl)
      }
    }
    n55 = Tick Count (ms)() -> (millisecond timer value=w44:u32)
    n56 = feedback #1(u32 0 ("millisecond timer value")) -> (w45:u32)
    n57 = feedback-in #1(w44) -> ()
    n58 = Subtract(x=w44, y=w45) -> (x-y=→"HENES Loop Time":u32)
    n59 = local read "Stop"() -> (w42:bool)
  }
  n60 = while {
    tunnel: w22 -> [w208]
    tunnel: "clustered_interpolator" ("function name") -> [w207]
    tunnel: [w206] -> w25
    tunnel: [w205] -> w26
    stop <- w209 stop-if-true
    # "클러스터링이랑 인터폴레이션 코드"
    # "Clustering"
    n61 = local read item#-1() -> (w187)
    n62 = local read "X_arrays_input"() -> (w204:i32[])
    n63 = local read "Y_arrays_input"() -> (w203:i32[])
    n64 = Tick Count (ms)() -> (millisecond timer value=w188:u32)
    n65 = node(w187, w208, w207, dbl[][] [] ("appended array"), w204, w203, "eps", "min_samples", "Threshold", "Spacing", "Ratio_Threshold") -> (w206:refnum<k35>, w205:errorcluster, w202:dbl[][])  [unwired: 8 in, 2 out]
    n66 = feedback #2(u32 0 ("millisecond timer value")) -> (w189:u32)
    n67 = feedback-in #2(w188) -> ()
    n68 = Index Array(array=w202) -> (element #1=w195:dbl[], element #2=w194:dbl[])  [unwired: 4 in]
    "X_arrays" <- w195
    "Y_arrays" <- w194
    n69 = Subtract(x=w188, y=w189) -> (x-y=→"PythonLoop":u32)
    n70 = Bundle("appended array"=w195, "appended array"=w194) -> (→"Clustered":T2)  [unwired: 1 in]
    n71 = Wait Until Next ms Multiple(millisecond multiple=u32 100) -> ()  [unwired: 1 out]
    n72 = local read "Stop"() -> (w209:bool)
  }
  n73 = while {
    tunnel: [w373] -> w40
    tunnel: [w374] -> w39
    tunnel: w31 -> [w382]
    tunnel: w30 -> [w381]
    shift-right: [w380] -> _
    shift-left: w29 -> [w383]
    stop <- "Stop" stop-if-true
    w238 = -450.0 ("element")
    w226 = 100.0 ("element")
    w228 = 450.0 ("element")
    w239 = 1200.0 ("f")
    w241 = 1200.0 ("element")
    w250 = dbl[] []
    w273 = 0.0 ("r")
    w309 = 0.0 ("element")
    w307 = -300.0 ("element")
    w310 = 800.0 ("element")
    w308 = 100.0 ("element")
    w311 = 450.0 ("element")
    w314 = 0.0 ("element")
    w312 = -300.0 ("element")
    w315 = -800.0 ("element")
    w313 = 100.0 ("element")
    w316 = -450.0 ("element")
    w349 = -800
    w350 = 800
    w351 = 700
    # "뒤로 빠꾸"
    # "사면초가면 Estop"
    # "배열에 inf가 2개 이상이면 중앙에 가까운 inf로 조향"
    # "예외처리를 안해서 좀 해야됨"
    # "더듬이로 길찾기"
    # "가까운 실제 존재 장애물은 피하기"
    # "전방만 감지"
    # "장애물 직교좌표계 포인트클라우드"
    # "RPLIDAR_S2를 통해 포인트 탐지 및 직교좌표계로 변환"
    # "Start Flag1 : A5\nStart Flag2 : 5A \nGET_HEALTH : A552"
    # "0번행렬 : x값\n1번행렬 : y값"
    # "중복점 제거 함수를 쓰기위해\n행렬을 전치하고 사용"
    # "Down-sampling(정수화)\n격자안에 포인트 1개만 넣기위해\n격자크기를 설정, 몫만 취하고 다시 원래 크기로 복원"
    # "Y"
    # "X"
    # "RPLIDAR_S2"
    n74 = local read "Stop"() -> (w379:bool)
    n75 = local read "X_arraysREAL"() -> (w216:i32[])
    n76 = local read "Y_arraysREAL"() -> (w215:i32[])
    n77 = Tick Count (ms)() -> (millisecond timer value=w378:u32)
    n78 = local read "X_arraysREAL"() -> (w217:i32[])
    n79 = local read "GoBack"() -> (w222:bool)
    n80 = local read "Y_arraysREAL"() -> (w218:i32[])
    n81 = case shown="2" w383 {
      tunnel: w382 -> [w531 w549 w572]
      tunnel: w381 -> [w530 w548 w571]
      tunnel: [w532 w545 w558] -> w380
      tunnel: [w521 w546 w574] -> w374
      tunnel: [w520 w547 w573] -> w373
      tunnel: w379 -> [_ _ w570]
      tunnel: ["" ("read buffer") w543 w569] -> w358
      frame 0, Default {
        w514 = u16 0 items=["GET_HEALTH", "SCAN_START", "Receive_Data"]
        w515 = u16 1 items=["GET_HEALTH", "SCAN_START", "Receive_Data"]
        n82 = VISA Write(VISA resource name=w531, write buffer="¥R", error in (no error)=w530) -> (VISA resource name out=w525:refnum<visa-resource-name>, error out=w524:errorcluster)  [unwired: 1 out]
        n83 = flat-sequence {
          tunnel: w525 -> [w534]
          tunnel: w524 -> [w533]
          tunnel: [w534] -> w523
          tunnel: [w533] -> w522
          frame #0 {
            n84 = Wait (ms)(milliseconds to wait=u32 5 ("대기 시간 (ms)")) -> ()  [unwired: 1 out]
          }
        }
        n85 = property class="Instr"(reference=w523, error in=w522) -> (reference out=w528:refnum<visa-resource-name>, error out=w527:errorcluster, "Serial Settings:Number of Bytes at Serial Port"=w526:u32)
        n86 = VISA Read(VISA resource name=w528, byte count=w526, error in (no error)=w527) -> (VISA resource name out=w520:refnum<visa-resource-name>, read buffer=w517:string, error out=w521:errorcluster)  [unwired: 1 out]
        n87 = Equal?(x=w517, y="¥Z\u0003\u0000\u0000\u0000\u0006\u0000\u0000\u0000") -> (x = y?=w518:bool)
        n88 = Select(t=w515, s=w518, f=w514) -> (s? t:f=w532:u16)
      }
      frame 1 {
        w536 = u16 2 items=["GET_HEALTH", "SCAN_START", "Receive_Data"]
        w537 = u16 1 items=["GET_HEALTH", "SCAN_START", "Receive_Data"]
        w550 = "¥Z\u0005\u0000\u0000@"
        n89 = VISA Write(VISA resource name=w549, write buffer="¥ \u0000", error in (no error)=w548) -> (VISA resource name out=w552:refnum<visa-resource-name>, error out=w553:errorcluster)  [unwired: 1 out]
        n90 = flat-sequence {
          tunnel: w552 -> [w556]
          tunnel: w553 -> [w555]
          tunnel: [w556] -> w539
          tunnel: [w555] -> w538
          frame #0 {
            n91 = Wait (ms)(milliseconds to wait=u32 5 ("대기 시간 (ms)")) -> ()  [unwired: 1 out]
          }
        }
        n92 = property class="Instr"(reference=w539, error in=w538) -> (reference out=w542:refnum<visa-resource-name>, error out=w541:errorcluster, "Serial Settings:Number of Bytes at Serial Port"=w540:u32)
        n93 = VISA Read(VISA resource name=w542, byte count=w540, error in (no error)=w541) -> (VISA resource name out=w547:refnum<visa-resource-name>, read buffer=w543:string, error out=w546:errorcluster)  [unwired: 1 out]
        n94 = Match Pattern(string=w543, regular expression=w550) -> (match substring=w544:string)  [unwired: 1 in, 3 out]
        n95 = Equal?(x=w544, y=w550) -> (x = y?=w554:bool)
        n96 = Select(t=w536, s=w554, f=w537) -> (s? t:f=w545:u16)
      }
      frame 2 {
        w558 = u16 2 items=["GET_HEALTH", "SCAN_START", "Receive_Data"]
        n97 = case shown="True" w570 {
          tunnel: w572 -> [w583 w587]
          tunnel: w571 -> [w582 w586]
          tunnel: [w583 w585] -> w568
          tunnel: [w582 w584] -> w567
          frame False {
          }
          frame True {
            n98 = VISA Write(VISA resource name=w587, write buffer="¥%", error in (no error)=w586) -> (VISA resource name out=w585:refnum<visa-resource-name>, error out=w584:errorcluster)  [unwired: 1 out]
          }
        }
        n99 = property class="Instr"(reference=w568, error in=w567) -> (reference out=w563:refnum<visa-resource-name>, error out=w562:errorcluster, "Serial Settings:Number of Bytes at Serial Port"=w564:u32)
        n100 = Greater?(x=w564, y=u32 8001) -> (0:w566:bool)
        n101 = case shown="True" w566 {
          tunnel: w563 -> [w576 w581]
          tunnel: w564 -> [_ w580]
          tunnel: w562 -> [w575 w579]
          tunnel: [w576 w578] -> w561
          tunnel: [w575 w577] -> w560
          frame False {
          }
          frame True {
            n102 = VISA Read(VISA resource name=w581, byte count=w580, error in (no error)=w579) -> (VISA resource name out=w578:refnum<visa-resource-name>, error out=w577:errorcluster)  [unwired: 2 out]
          }
        }
        n103 = VISA Read(VISA resource name=w561, byte count=u32 8000, error in (no error)=w560) -> (VISA resource name out=w573:refnum<visa-resource-name>, read buffer=w569:string, error out=w574:errorcluster)  [unwired: 1 out]
      }
    }
    "read buffer" <- w358
    n104 = feedback #3(u32 0 ("millisecond timer value")) -> (w377:u32)
    n105 = feedback-in #3(w378) -> ()
    n106 = Select(t=1700.0, s=w222, f=950.0 ("element")) -> (s? t:f=w220:dbl)
    n107 = local read "X_arraysREAL"() -> (w232:i32[])
    n108 = local read "Y_arraysREAL"() -> (w233:i32[])
    n109 = Subtract(x=w378, y=w377) -> (x-y=→"LidarLoop":u32)
    n110 = Build Array(w316, w316, w315, w315, w314, w314, w316) -> (w332:dbl[])
    n111 = Build Array(w313, w312, w312, w241, w241, w313, w313) -> (w333:dbl[])
    n112 = Build Array(w311, w311, w310, w310, w309, w309, w311) -> (w340:dbl[])
    n113 = Build Array(w308, w307, w307, w239, w239, w308, w308) -> (w339:dbl[])
    n114 = Build Array(w228, w228, w238, w238, w228) -> (w230:dbl[])
    n115 = Build Array(w226, w220, w220, w226, w226) -> (w231:dbl[])
    n116 = call "ROI_IN_Check.vi"("도형Y좌표"=w333, "도형X좌표"=w332, "LiDAR_Y"=w218, "LiDAR_X"=w217) -> ("ROI_IN_Y"=w330:i32[], "ROI_IN_X"=w331:i32[])  [unwired: 6 in]
    n117 = Bundle(w332, w333) -> (→"NearCarROILeft":cluster{dbl[], dbl[]})  [unwired: 1 in]
    n118 = call "ROI_IN_Check.vi"("도형Y좌표"=w339, "도형X좌표"=w340, "LiDAR_Y"=w215, "LiDAR_X"=w216) -> ("ROI_IN_Y"=w327:i32[], "ROI_IN_X"=w328:i32[])  [unwired: 6 in]
    n119 = Bundle(w340, w339) -> (→"NearCarROIRight":cluster{dbl[], dbl[]})  [unwired: 1 in]
    n120 = call "ROI_IN_Check.vi"("도형Y좌표"=w231, "도형X좌표"=w230, "LiDAR_Y"=w233, "LiDAR_X"=w232) -> ("ROI_IN_Y"=w236:i32[], "ROI_IN_X"=w235:i32[])  [unwired: 6 in]
    n121 = Bundle(w230, w231) -> (→"GobackROI":cluster{dbl[], dbl[]})  [unwired: 1 in]
    n122 = Wait Until Next ms Multiple(millisecond multiple=u32 100) -> ()  [unwired: 1 out]
    n123 = Bundle("ROI_IN_X"=w331, "ROI_IN_Y"=w330) -> (→"NearCarPointsLeft":cluster{"ROI_IN_X":i32[], "ROI_IN_Y":i32[]})  [unwired: 1 in]
    n124 = Bundle("ROI_IN_X"=w328, "ROI_IN_Y"=w327) -> (→"NearCarPointsRight":cluster{"ROI_IN_X":i32[], "ROI_IN_Y":i32[]})  [unwired: 1 in]
    n125 = Re/Im To Polar(2:w330, 3:w331) -> (1:w329:dbl[])  [unwired: 1 out]
    n126 = Re/Im To Polar(2:w327, 3:w328) -> (1:w326:dbl[])  [unwired: 1 out]
    n127 = Re/Im To Polar(2:w236, 3:w235) -> (1:w237:dbl[])  [unwired: 1 out]
    n128 = Array Max & Min(array=w329) -> (min value=w325:dbl)  [unwired: 3 out]
    n129 = Array Size(array=w329) -> (size(s)=w334:i32)
    n130 = Array Max & Min(array=w326) -> (min value=w324:dbl)  [unwired: 3 out]
    n131 = Array Size(array=w326) -> (size(s)=w341:i32)
    n132 = Array Size(array=w237) -> (size(s)=w229:i32)
    n133 = Divide(x=40000.0, y=w325) -> (x/y=w322:dbl)
    "NearLeft" <- w322
    n134 = Not Equal To 0?(x=w334) -> (x != 0?=w317:bool)
    "Too Close" <- w317
    n135 = Divide(x=-40000.0, y=w324) -> (x/y=w320:dbl)
    "NearRight" <- w320
    n136 = Not Equal To 0?(x=w341) -> (x != 0?=w318:bool)
    "Too Close" <- w318
    n137 = Not Equal To 0?(x=w229) -> (x != 0?=w225:bool)
    n138 = local write "GoBack"(w225) -> ()
    n139 = Select(t=w322, s=w317, f=0.0) -> (s? t:f=w321:dbl)
    n140 = Select(t=w320, s=w318, f=0.0) -> (s? t:f=w319:dbl)
    n141 = Or(x=w317, y=w318) -> (x .or. y?=→"TooClose":bool)
    n142 = Add(x=w321, y=w319) -> (x+y=→"NearSteer":dbl)
    n143 = local read "X_arrays"() -> (w306:dbl[])
    n144 = local read "Y_arrays"() -> (w305:dbl[])
    n145 = call "PRLIDAR_5byte_Pasing.vi"("RPLIDAR_Data"=w358) -> ("Theta(deg)"=w361:dbl[], "Distance(mm)"=w362:dbl[])  [unwired: 9 in]
    n146 = call "RPLiDAR_축변환.vi"("Distance(mm)"=w361, "Theta(deg)"=w362) -> ("Y"=w359:dbl[], "X"=w360:dbl[])  [unwired: 8 in]
    n147 = for {
      tunnel: w360 -> [w513] mode=indexing
      tunnel: w359 -> [w512] mode=indexing
      tunnel: [w509] -> w371 mode=indexing
      tunnel: [w508] -> w372 mode=indexing
      n148 = Quotient & Remainder(x=w513, y="격자크기") -> (floor(x/y)=w511:dbl)  [unwired: 1 out]
      n149 = Quotient & Remainder(x=w512, y="격자크기") -> (floor(x/y)=w510:dbl)  [unwired: 1 out]
      n150 = Multiply(x=w511, y="격자크기") -> (x*y=w509:dbl)
      n151 = Multiply(x=w510, y="격자크기") -> (x*y=w508:dbl)
    }
    n152 = Re/Im To Polar(2:w305, 3:w306) -> (0:w304:dbl[], 1:w303:dbl[])
    n153 = for {
      tunnel: w304 -> [w506] mode=indexing
      tunnel: w303 -> [w428] mode=indexing
      shift-right: [w473] -> w302
      shift-left: w250 -> [w405]
      shift-right: [w472] -> w301
      shift-left: w250 -> [w406]
      shift-right: [w471] -> w300
      shift-left: w250 -> [w407]
      shift-right: [w470] -> w299
      shift-left: w250 -> [w408]
      shift-right: [w469] -> w298
      shift-left: w250 -> [w409]
      shift-right: [w468] -> w297
      shift-left: w250 -> [w410]
      shift-right: [w467] -> w296
      shift-left: w250 -> [w411]
      shift-right: [w466] -> w295
      shift-left: w250 -> [w412]
      shift-right: [w462] -> w289
      shift-left: w250 -> [w413]
      shift-right: [w426] -> w258
      shift-left: w250 -> [w414]
      shift-right: [w425] -> w257
      shift-left: w250 -> [w415]
      shift-right: [w424] -> w256
      shift-left: w250 -> [w416]
      shift-right: [w423] -> w255
      shift-left: w250 -> [w417]
      shift-right: [w419] -> w251
      shift-left: w250 -> [w401]
      shift-right: [w420] -> w252
      shift-left: w250 -> [w402]
      shift-right: [w421] -> w253
      shift-left: w250 -> [w403]
      shift-right: [w422] -> w254
      shift-left: w250 -> [w404]
      w427 = inf
      n154 = expression code="(x/pi)*180.0" "radians to degrees"(w506) -> (w446:dbl)
      n155 = In Range and Coerce(upper limit=177.5, x=w446, lower limit=162.5) -> (In Range?=w433:bool)  [unwired: 1 out]
      n156 = In Range and Coerce(upper limit=167.5, x=w446, lower limit=152.5 ("upper limit")) -> (In Range?=w434:bool)  [unwired: 1 out]
      n157 = In Range and Coerce(upper limit=157.5 ("lower limit"), x=w446, lower limit=142.5 ("upper limit")) -> (In Range?=w435:bool)  [unwired: 1 out]
      n158 = In Range and Coerce(upper limit=147.5 ("lower limit"), x=w446, lower limit=132.5 ("upper limit")) -> (In Range?=w436:bool)  [unwired: 1 out]
      n159 = In Range and Coerce(upper limit=137.5, x=w446, lower limit=122.5) -> (In Range?=w487:bool)  [unwired: 1 out]
      n160 = In Range and Coerce(upper limit=127.5, x=w446, lower limit=112.5) -> (In Range?=w489:bool)  [unwired: 1 out]
      n161 = In Range and Coerce(upper limit=117.5, x=w446, lower limit=102.5) -> (In Range?=w485:bool)  [unwired: 1 out]
      n162 = In Range and Coerce(upper limit=112.5, x=w446, lower limit=90.0) -> (In Range?=w484:bool)  [unwired: 1 out]
      n163 = In Range and Coerce(upper limit=97.5, x=w446, lower limit=82.5) -> (In Range?=w483:bool)  [unwired: 1 out]
      n164 = In Range and Coerce(upper limit=90.0, x=w446, lower limit=67.5) -> (In Range?=w482:bool)  [unwired: 1 out]
      n165 = In Range and Coerce(upper limit=77.5, x=w446, lower limit=62.5) -> (In Range?=w481:bool)  [unwired: 1 out]
      n166 = In Range and Coerce(upper limit=67.5, x=w446, lower limit=52.5) -> (In Range?=w480:bool)  [unwired: 1 out]
      n167 = In Range and Coerce(upper limit=57.5, x=w446, lower limit=42.5) -> (In Range?=w465:bool)  [unwired: 1 out]
      n168 = In Range and Coerce(upper limit=47.5, x=w446, lower limit=32.5) -> (In Range?=w444:bool)  [unwired: 1 out]
      n169 = In Range and Coerce(upper limit=37.5, x=w446, lower limit=22.5) -> (In Range?=w443:bool)  [unwired: 1 out]
      n170 = In Range and Coerce(upper limit=27.5, x=w446, lower limit=12.5) -> (In Range?=w442:bool)  [unwired: 1 out]
      n171 = In Range and Coerce(upper limit=17.5, x=w446, lower limit=2.5) -> (In Range?=w441:bool)  [unwired: 1 out]
      n172 = Select(t=w428, s=w433, f=w427) -> (s? t:f=w432:dbl)
      n173 = Select(t=w428, s=w434, f=w427) -> (s? t:f=w431:dbl)
      n174 = Select(t=w428, s=w435, f=w427) -> (s? t:f=w430:dbl)
      n175 = Select(t=w428, s=w436, f=w427) -> (s? t:f=w429:dbl)
      n176 = Select(t=w428, s=w487, f=w427) -> (s? t:f=w486:dbl)
      n177 = Select(t=w428, s=w489, f=w427) -> (s? t:f=w488:dbl)
      n178 = Select(t=w428, s=w485, f=w427) -> (s? t:f=w474:dbl)
      n179 = Select(t=w428, s=w484, f=w427) -> (s? t:f=w475:dbl)
      n180 = Select(t=w428, s=w483, f=w427) -> (s? t:f=w476:dbl)
      n181 = Select(t=w428, s=w482, f=w427) -> (s? t:f=w477:dbl)
      n182 = Select(t=w428, s=w481, f=w427) -> (s? t:f=w478:dbl)
      n183 = Select(t=w428, s=w480, f=w427) -> (s? t:f=w479:dbl)
      n184 = Select(t=w428, s=w465, f=w427) -> (s? t:f=w445:dbl)
      n185 = Select(t=w428, s=w444, f=w427) -> (s? t:f=w440:dbl)
      n186 = Select(t=w428, s=w443, f=w427) -> (s? t:f=w439:dbl)
      n187 = Select(t=w428, s=w442, f=w427) -> (s? t:f=w438:dbl)
      n188 = Select(t=w428, s=w441, f=w427) -> (s? t:f=w437:dbl)
      n189 = Insert Into Array(array=w401, new element=w432) -> (w419:dbl[])  [unwired: 1 in]
      n190 = Insert Into Array(array=w402, new element=w431) -> (w420:dbl[])  [unwired: 1 in]
      n191 = Insert Into Array(array=w403, new element=w430) -> (w421:dbl[])  [unwired: 1 in]
      n192 = Insert Into Array(array=w404, new element=w429) -> (w422:dbl[])  [unwired: 1 in]
      n193 = Insert Into Array(array=w405, new element=w486) -> (w473:dbl[])  [unwired: 1 in]
      n194 = Insert Into Array(array=w406, new element=w488) -> (w472:dbl[])  [unwired: 1 in]
      n195 = Insert Into Array(array=w407, new element=w474) -> (w471:dbl[])  [unwired: 1 in]
      n196 = Insert Into Array(array=w408, new element=w475) -> (w470:dbl[])  [unwired: 1 in]
      n197 = Insert Into Array(array=w409, new element=w476) -> (w469:dbl[])  [unwired: 1 in]
      n198 = Insert Into Array(array=w410, new element=w477) -> (w468:dbl[])  [unwired: 1 in]
      n199 = Insert Into Array(array=w411, new element=w478) -> (w467:dbl[])  [unwired: 1 in]
      n200 = Insert Into Array(array=w412, new element=w479) -> (w466:dbl[])  [unwired: 1 in]
      n201 = Insert Into Array(array=w413, new element=w445) -> (w462:dbl[])  [unwired: 1 in]
      n202 = Insert Into Array(array=w414, new element=w440) -> (w426:dbl[])  [unwired: 1 in]
      n203 = Insert Into Array(array=w415, new element=w439) -> (w425:dbl[])  [unwired: 1 in]
      n204 = Insert Into Array(array=w416, new element=w438) -> (w424:dbl[])  [unwired: 1 in]
      n205 = Insert Into Array(array=w417, new element=w437) -> (w423:dbl[])  [unwired: 1 in]
    }
    n206 = To Long Integer(number=w371) -> (32bit integer=w366:i32[])
    n207 = To Long Integer(number=w372) -> (32bit integer=w365:i32[])
    n208 = Build Array(w366, w365) -> (w367:i32[][])
    n209 = Transpose 2D Array(2D array=w367) -> (transposed array=w363:i32[][])
    n210 = call "Remove Duplicates From 1D Array.vim"("array"=w363) -> ("array with duplicates removed"=w364:i32[][])  [unwired: 10 in]
    n211 = Negate(x=w351) -> (-x=w354:i32)
    n212 = Transpose 2D Array(2D array=w364) -> (transposed array=w368:i32[][])
    n213 = Negate(x="Looking X") -> (-x=w355:i32)
    n214 = Index Array(array=w368, index (row) #1=0 ("index (row)"), index (row) #2=1 ("index (row)")) -> (element #1=w343:i32[], element #2=w342:i32[])  [unwired: 2 in]
    "X_arraysREAL" <- w343
    "Y_arraysREAL" <- w342
    n215 = Build Array(w351, w351, "Looking X", "Looking X", w355, w355, w354, w354, w351) -> (w348:i32[])
    n216 = Build Array(w350, w349, w349, "Looking Y", "Looking Y", w349, w349, w350, w350) -> (w347:i32[])
    n217 = Array Max & Min(array=w251) -> (min value=w243:dbl)  [unwired: 3 out]
    n218 = Array Max & Min(array=w252) -> (min value=w245:dbl)  [unwired: 3 out]
    n219 = Array Max & Min(array=w253) -> (min value=w247:dbl)  [unwired: 3 out]
    n220 = Array Max & Min(array=w254) -> (min value=w249:dbl)  [unwired: 3 out]
    n221 = Array Max & Min(array=w302) -> (min value=w280:dbl)  [unwired: 3 out]
    n222 = Array Max & Min(array=w301) -> (min value=w282:dbl)  [unwired: 3 out]
    n223 = Array Max & Min(array=w300) -> (min value=w284:dbl)  [unwired: 3 out]
    n224 = Array Max & Min(array=w299) -> (min value=w286:dbl)  [unwired: 3 out]
    n225 = Array Max & Min(array=w298) -> (min value=w212:dbl)  [unwired: 3 out]
    n226 = Array Max & Min(array=w297) -> (min value=w285:dbl)  [unwired: 3 out]
    n227 = Array Max & Min(array=w296) -> (min value=w283:dbl)  [unwired: 3 out]
    n228 = Array Max & Min(array=w295) -> (min value=w281:dbl)  [unwired: 3 out]
    n229 = Array Max & Min(array=w289) -> (min value=w279:dbl)  [unwired: 3 out]
    n230 = Array Max & Min(array=w258) -> (min value=w248:dbl)  [unwired: 3 out]
    n231 = Array Max & Min(array=w257) -> (min value=w246:dbl)  [unwired: 3 out]
    n232 = Array Max & Min(array=w256) -> (min value=w244:dbl)  [unwired: 3 out]
    n233 = Array Max & Min(array=w255) -> (min value=w242:dbl)  [unwired: 3 out]
    n234 = call "ROI_IN_Check.vi"("도형Y좌표"=w347, "도형X좌표"=w348, "LiDAR_Y"=w342, "LiDAR_X"=w343) -> ("ROI_IN_Y"=→"Y_arrays_input":i32[], "ROI_IN_X"=→"X_arrays_input":i32[])  [unwired: 6 in]
    n235 = Less?(x=w212, y=3000.0) -> (x < y?=w213:bool)
    n236 = Bundle(w348, w347) -> (→"LookingAt":cluster{i32[], i32[]})  [unwired: 1 in]
    n237 = Select(t=w212, s=w213, f=inf) -> (s? t:f=w211:dbl)
    n238 = Build Array(w211, w286, w285, w284, w283, w282, w281, w280, w279, w249, w248, w247, w246, w245, w244, w243, w242) -> (w287:dbl[])
    n239 = Array Max & Min(array=w287) -> (max value=w240:dbl, max index (indices)=w278:i32)  [unwired: 2 out]
    n240 = case shown="7" w278 {
      tunnel: [90.0 100.0 80.0 110.0 70.0 120.0 60.0 130.0 50.0 140.0 40.0 150.0 30.0 160.0 20.0 170.0 10.0] -> w277
      frame 0, Default {
      }
      frame 1 {
      }
      frame 2 {
      }
      frame 3 {
      }
      frame 4 {
      }
      frame 5 {
      }
      frame 6 {
      }
      frame 7 {
      }
      frame 8 {
      }
      frame 9 {
      }
      frame 10 {
      }
      frame 11 {
      }
      frame 12 {
      }
      frame 13 {
      }
      frame 14 {
      }
      frame 15 {
      }
      frame 16 {
      }
    }
    n241 = Less?(x=w240, y="length") -> (x < y?=→"VEstop":bool)
    n242 = local read "NearCarPointsRight"() -> (w269:cluster{"ROI_IN_X":dbl[], "ROI_IN_Y":dbl[]})
    n243 = local read "NearCarPointsLeft"() -> (w266:cluster{"ROI_IN_X":dbl[], "ROI_IN_Y":dbl[]})
    n244 = local read "NearCarROIRight"() -> (w270:cluster{i32[], i32[]})
    n245 = local read "TargetDerection"() -> (w264:cluster{dbl[], dbl[]})
    n246 = local read "NearCarROILeft"() -> (w267:cluster{i32[], i32[]})
    n247 = local read "GobackROI"() -> (w227:cluster{i32[], i32[]})
    n248 = local read "LookingAt"() -> (w265:cluster{i32[], i32[]})
    n249 = local read "Clustered"() -> (w271:T2)
    n250 = Negate(x=w277) -> (-x=w276:dbl)
    n251 = Add(x=90.0, y=w276) -> (x+y=→"Anthena_Steer":dbl)
    n252 = Build Array(w265, w266, w267, w269, w270, w271, w264, w227) -> (→"PointCloud":T1)
    n253 = expression code="(x/180.0)*pi" "degrees to radians"(w277) -> (w288:dbl)
    n254 = Polar To Re/Im(2:w288, 3:7000.0 ("r")) -> (0:w293:dbl, 1:w294:dbl)
    n255 = Build Array(w294, w273) -> (w292:dbl[])
    n256 = Build Array(w293, w273) -> (w291:dbl[])
    n257 = Bundle(w292, w291) -> (→"TargetDerection":cluster{dbl[], dbl[]})  [unwired: 1 in]
  }
  n258 = while {
    stop <- w590 stop-if-true
    # "Controller"
    n259 = local read "VEstop"() -> (w589:bool)
    n260 = case shown="False" w589 {
      frame False {
        n261 = case shown="False" "GoBack" {
          frame False {
            n262 = local read "TooClose"() -> (w593:bool)
            n263 = local write "HLV_Gear"(u8 0 ("HLV_Gear")) -> ()
            n264 = expression code="x/(0.00001*27*pi*60)"("Input_Spd(kph)") -> (w598:dbl)
            n265 = case shown="False" w593 {
              tunnel: [w604 w616] -> w592
              frame False {
                n266 = local read "Anthena_Steer"() -> (w613:i32)
                n267 = local read item#-1() -> (w610)
                n268 = Absolute Value(x=w610) -> (abs(x)=w611:dbl)
                n269 = Multiply(x=w610, y=w613) -> (x*y=w615:i32)
                n270 = Equal?(x=w613, y=0) -> (x = y?=w612:bool)
                n271 = Less?(x=w611, y=30.0) -> (x < y?=w609:bool)
                n272 = Greater?(x=w615, y=0.0) -> (0:w614:bool)
                n273 = local read item#-1() -> (w603)
                n274 = And(x=w609, y=w612) -> (x .and. y?=w608:bool)
                n275 = Or(x=w614, y=w608) -> (x .or. y?=w602:bool)
                n276 = Or(x=w603, y=w602) -> (x .or. y?=w601:bool)
                n277 = Select(t=w610, s=w601, f=w613) -> (s? t:f=w604:i32)
              }
              frame True {
                n278 = local read "NearSteer"() -> (w616:dbl)
              }
            }
            n279 = expression code="x*4.35*1.8"(w598) -> (w595:dbl)
            n280 = Multiply(x=0.5, y=w595) -> (x*y=w596:dbl)
            n281 = Select(t=w596, s=w593, f=w595) -> (s? t:f=→"Input_Spd(cmd)":dbl)
            n282 = local write "InputSteer(cmd)"(w592) -> ()
          }
          frame True {
            n283 = flat-sequence {
              frame #0 {
                n284 = Wait (ms)(milliseconds to wait=u32 1000) -> ()  [unwired: 1 out]
                n285 = local write "InputSteer(cmd)"(0.0 ("InputSteer(cmd)")) -> ()
              }
              frame #1 {
                n286 = local write "HLV_Gear"(u8 2 ("HLV_Gear")) -> ()
              }
              frame #2 {
                n287 = while {
                  stop <- w622 continue-if-true
                  n288 = expression code="x/(0.00001*27*pi*60)"(6.0 ("Input_Spd(kph)")) -> (w625:dbl)
                  n289 = local read "NearSteer"() -> (w620:dbl)
                  n290 = Negate(x=w620) -> (-x=w621:dbl)
                  n291 = expression code="x*4.35*1.8"(w625) -> (w623:dbl)
                  n292 = local read "GoBack"() -> (w622:bool)
                  n293 = local write "Input_Spd(cmd)"(w621) -> ()
                  n294 = local write "Input_Spd(cmd)"(w623) -> ()
                }
              }
              frame #3 {
                w627 = 0.0 ("InputSteer(cmd)")
                n295 = Wait (ms)(milliseconds to wait=u32 1000) -> ()  [unwired: 1 out]
                n296 = local write "InputSteer(cmd)"(w627) -> ()
                n297 = local write "Input_Spd(cmd)"(w627) -> ()
              }
            }
          }
        }
      }
      frame True {
        n298 = local write "Input_Spd(cmd)"(0.0 ("Input_Spd(cmd)")) -> ()
      }
    }
    n299 = local read "Stop"() -> (w590:bool)
  }
  n300 = Close Python Session(session in=w25, error in=w26) -> (11:→"Clustering Error":errorcluster)
  n301 = VISA Flush I/O Buffer(VISA resource name=w16, error in (no error)=w15) -> (VISA resource name out=w19:refnum<visa-resource-name>, error out=w20:errorcluster)  [unwired: 1 in]
  n302 = VISA Close(VISA resource name=w19, error in (no error)=w20) -> (error out=w14:errorcluster)
  n303 = call <vilib>:"Simple Error Handler.vi"("error in (no error)"=w14) -> ()  [unwired: 4 in, 5 out]
  n304 = VISA Close(VISA resource name=w40, error in (no error)=w39) -> (error out=w41:errorcluster)
  n305 = call <vilib>:"Clear Errors.vi"("error in (no error)"=w41) -> ()  [unwired: 5 in, 2 out]
